vi "Read VBAI Para.vi"(8 "error in (no error)":errorcluster, 11 "Fiber Auto Collimation state data in":refnum<class "Fiber Auto Collimation state data.lvclass">) -> (0 "error out":errorcluster, 2 "VBAI":cluster{"New Image":T1, "VBAI Session Out":T2}, 3 "Fiber Auto Collimation state data out":refnum<class "Fiber Auto Collimation state data.lvclass">)   [LabVIEW 2018, in "Fiber Auto Collimation state data.lvclass"]
doc: "Serial number of the Device Under Test."
uses:
  Fiber Auto Collimation state data.lvclass
  <vilib>/vision/Image Controls.llb/IMAQ Image.ctl
  <vilib>/userdefined/High Color/VBAIInterface.ctl
  Fiber Auto Collimation state data.lvclass/Fiber Auto Collimation state data.ctl
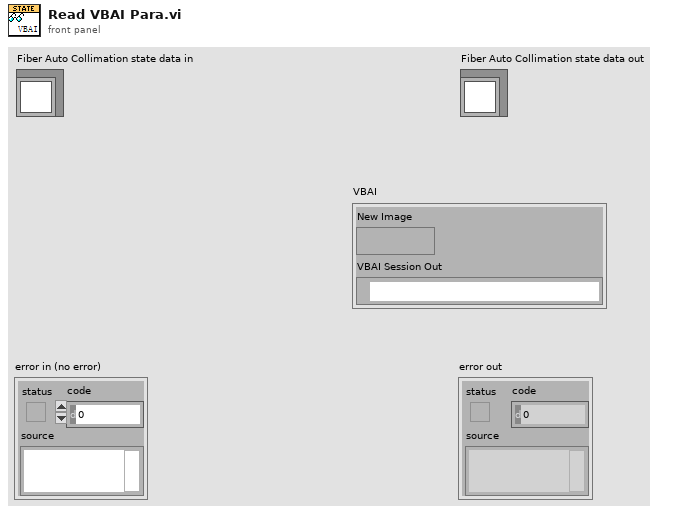
[diagram p1: front panel]
types:
  T1 = typedef "IMAQ Image.ctl" = refnum<image>
  T2 = typedef "VBAIInterface.ctl" = refnum<k21>
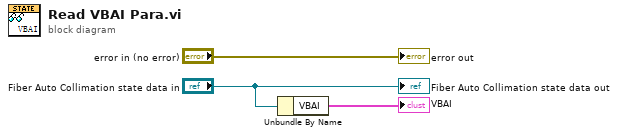
[diagram p0: block diagram]
diagram:
  n1 = Unbundle By Name("Fiber Auto Collimation state data in") -> ("VBAI"=→"VBAI":cluster{"New Image":T1, "VBAI Session Out":T2})
  "error out" <- "error in (no error)"
  "Fiber Auto Collimation state data out" <- "Fiber Auto Collimation state data in"
